vi "Factory_Acceptance_Test.vi"() -> ()   [LabVIEW 2020]
uses:
  <vilib>/Retry/UI Control Suite/Boolean/System Buttons/Graph Button.ctl
  Driver/E5071C/E5071C/E5071C.lvclass
  Driver/PEU/PEU/PEU.lvclass
  <vilib>/Utility/NIReport.llb/Report Type.ctl
  Driver/E5071C/E5071C/E5071C.lvclass/E5071C.ctl
  <vilib>/addons/_office/excel.llb/Excel Get Data ([str]).vi
  <vilib>/addons/_office/excel.llb/Excel Easy Table (str).vi
  <vilib>/Utility/NIReport.llb/NI_report.lvclass
  <instrlib>/Agilent ENA Series/Agilent ENA Series.lvlib
  <vilib>/Utility/NIReport.llb/NI_ReportGenerationCore.lvlib
  <vilib>/Utility/NIReport.llb/Excel/NI_Excel.lvclass
  <vilib>/addons/_office/NI_ReportGenerationToolkit.lvlib
panel:
  in  "Load":bool
  in  "Test":bool
  in  "Save":bool
  in  "负载选择":enum32{"Item 0", "Item 1"}(radio)
  in  "Limit Line":T1
  in  "DUT ID:":string
  in  "DUT\n开关类型":string(combo)="SPDT"
  in  "Panel Show":bool
  in  "Tab Control":enum32{"驻波VSWR", "插入损耗IL", "隔离度ISL"}(tab)
  out "VSWR_State":string
  out "VSWR Graph":cluster{"频率":dbl[], dbl[]}[](graph)
  out "IL_State":string
  out "IL Graph":cluster{"Freqs":dbl[], "temp_value":dbl[]}[](graph)
  out "ISL_State":string
  out "ISL Graph":cluster{"Freqs":dbl[], "temp_value":dbl[]}[](graph)
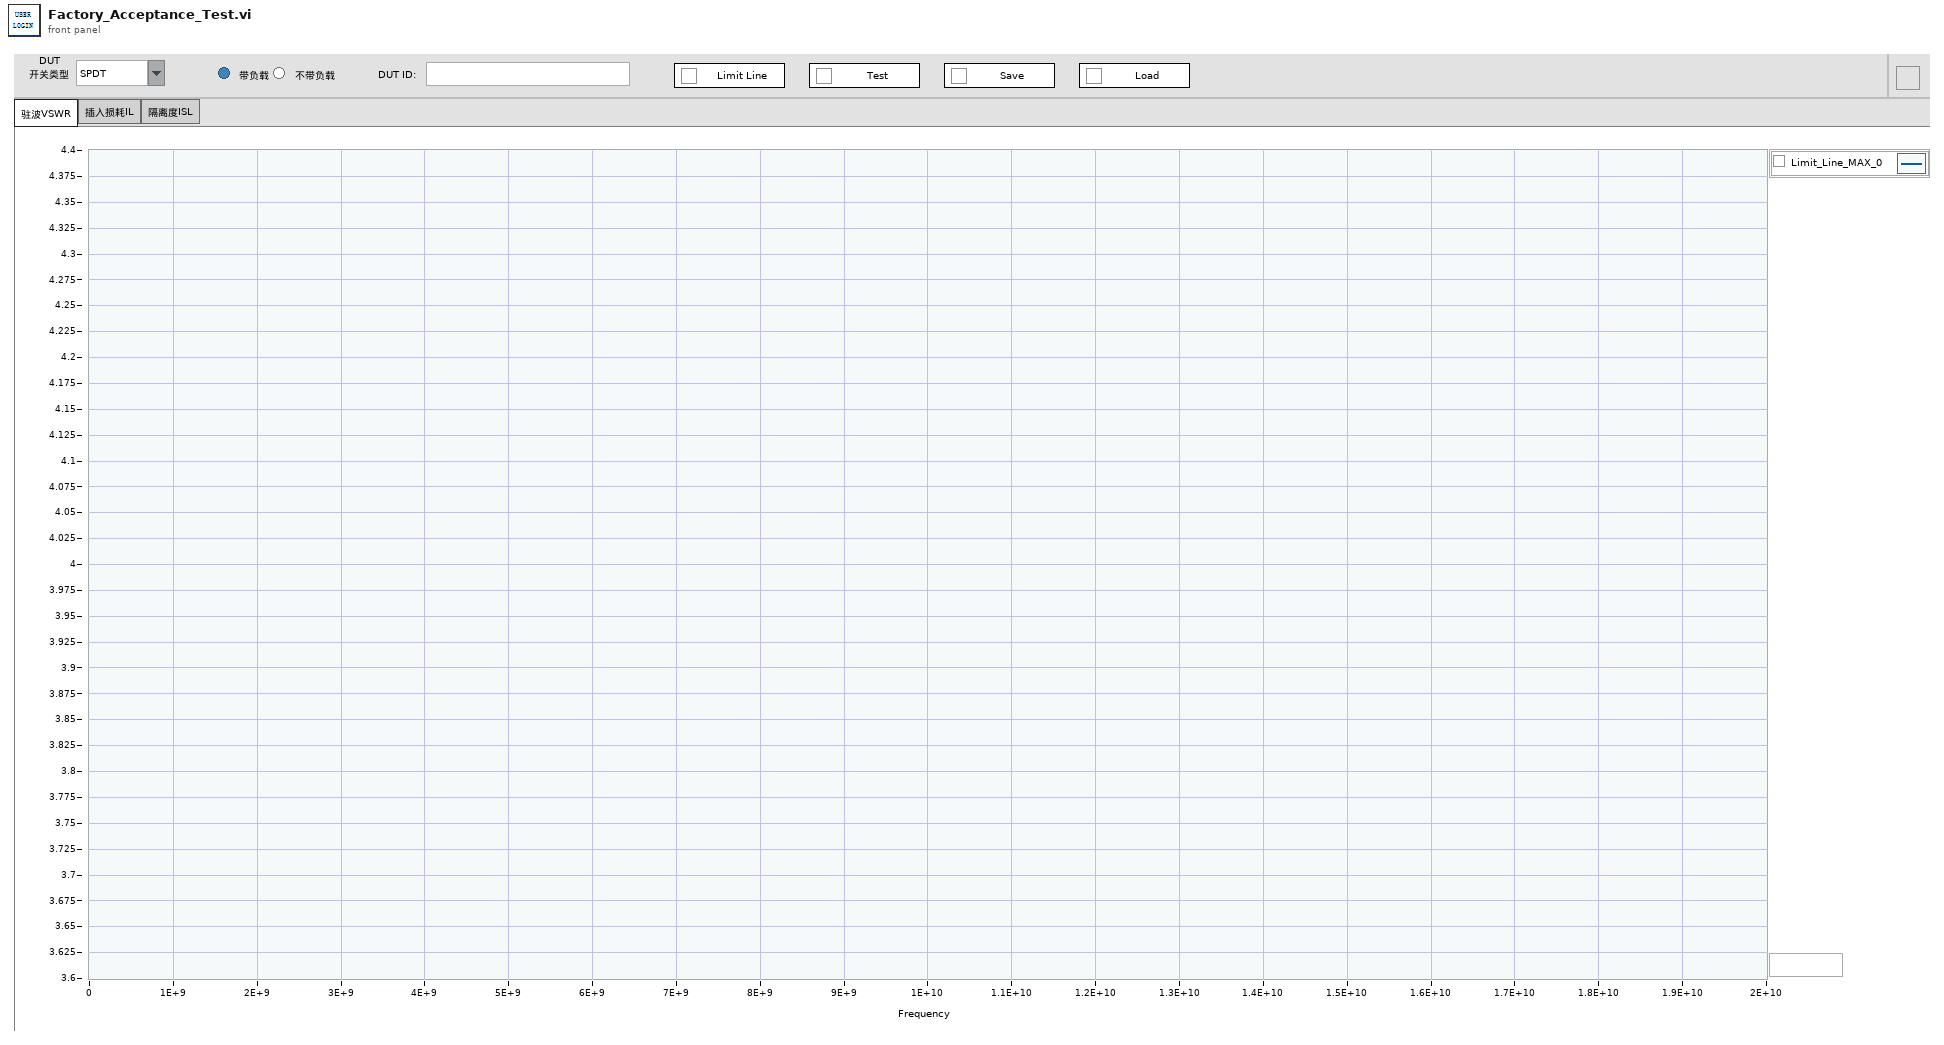
[diagram p1: front panel]
types:
  T1 = typedef "Graph Button.ctl" = bool
  T2 = enum32{"Invalid", "Standard", "Closed", "Hidden", "Minimized", "Maximized"}
  T3 = cluster{"Limit_IL":string[][], "Limit_VSWR":string[][], "Limit_ISL":string[][]}
  T4 = cluster{"校准文件":string[], "控制箱通道":string[], "DUT导通引脚":string[], "S名称":string[], "配置S":string[], "Plot_Name":string[]}
  T5 = typedef "NI_ReportGenerationCore.lvlib/Report Type.ctl" = enum16{"HTML", "Word", "Excel"}
  T6 = enum16{"maximized", "minimized", "normal", "no change"}
  T7 = cluster{"E5071C":refnum<class "E5071C.lvclass">, "PEU":refnum<class "PEU.lvclass">, "Index":i32, "Limit_Table":cluster{"Limit_IL":string[][], "Limit_VSWR":string[][], "Limit_ISL":string[][]}, "VSWR Graph":cluster{"频率":dbl[], dbl[]}[], "temp_value":dbl[], "Freqs":dbl[], "Count":i32, "测试逻辑":cluster{"校准文件":string[], "控制箱通道":string[], "DUT导通引脚":string[], "S名称":string[], "配置S":string[], "Plot_Name":string[]}, "VSWR_State":bool, "IL_State":bool, "ISL_State":bool, "Limit_Line_State":bool}
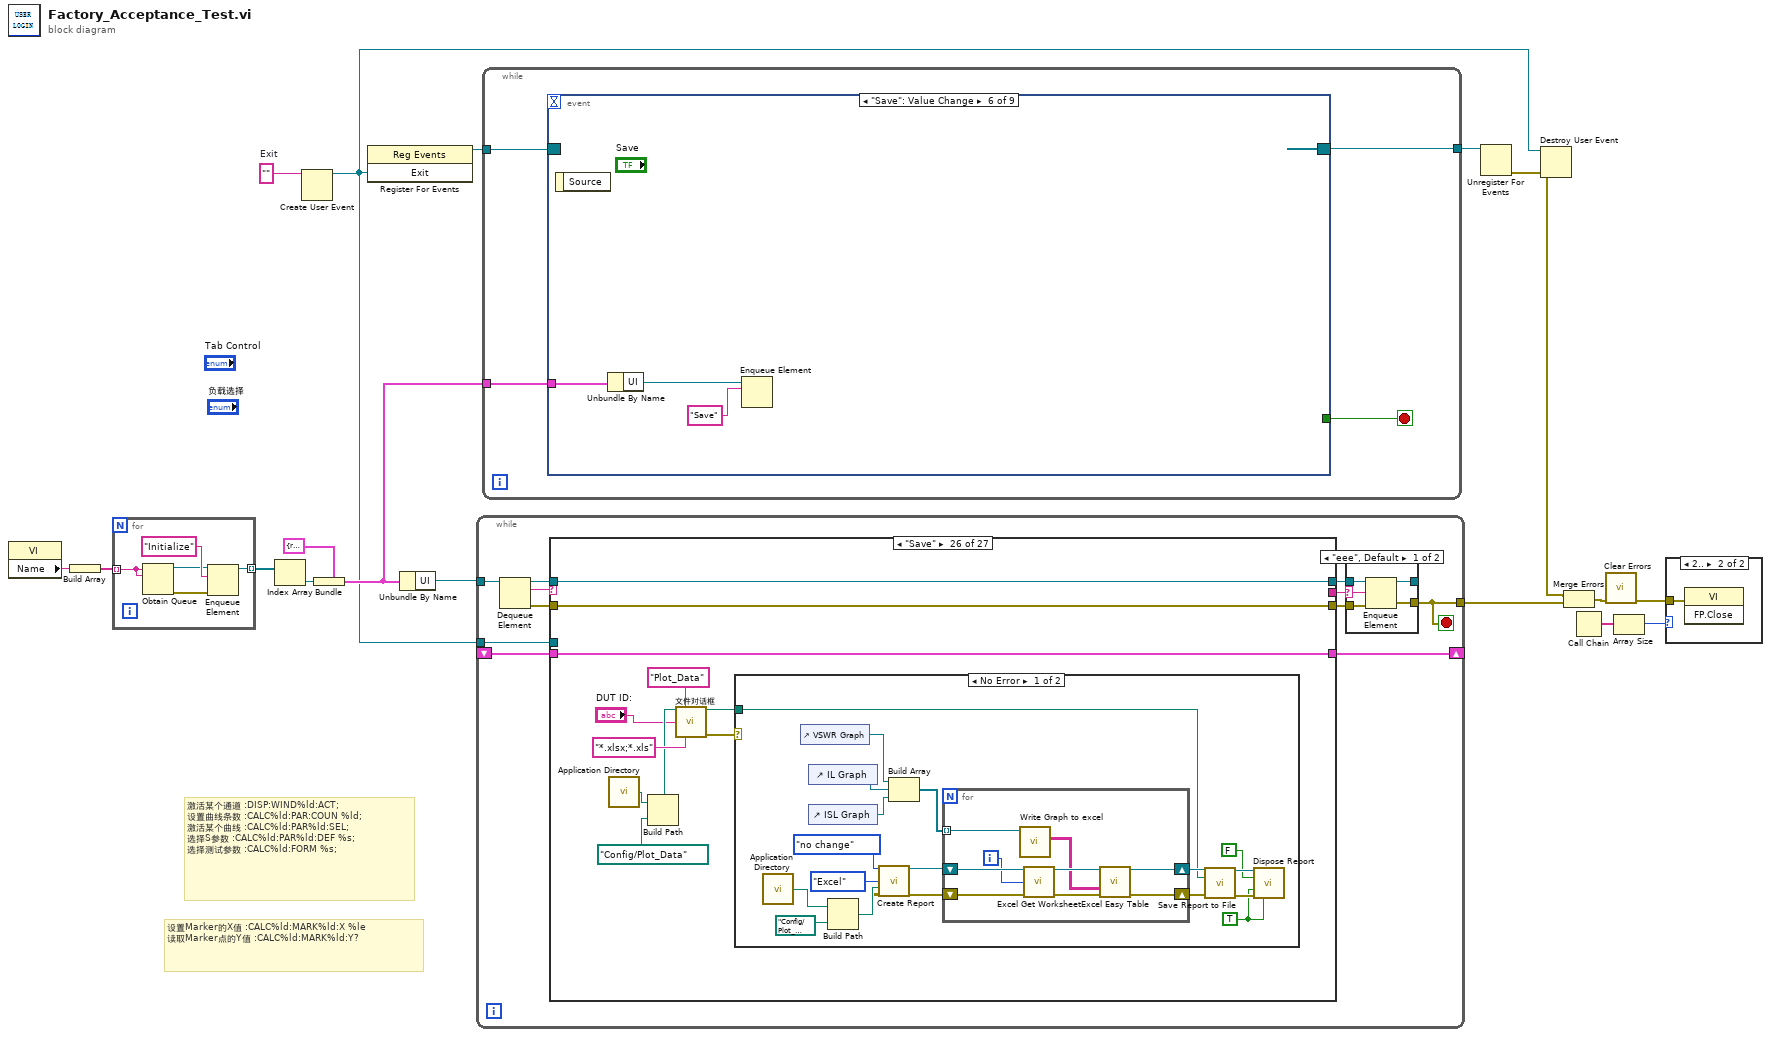
[diagram p0: block diagram]
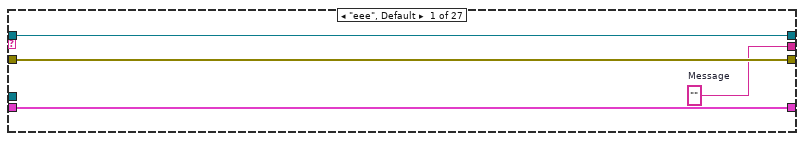
[diagram p4: hidden frame]
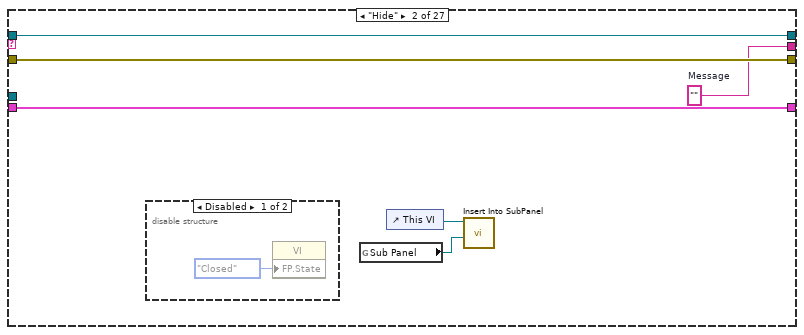
[diagram p5: hidden frame]
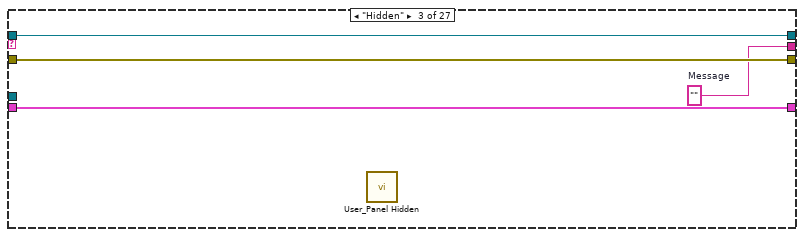
[diagram p7: hidden frame]
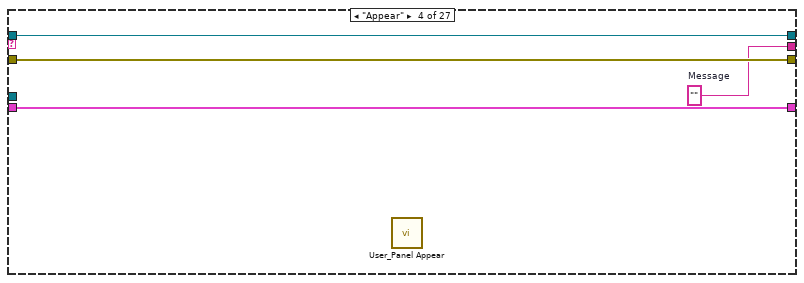
[diagram p8: hidden frame]
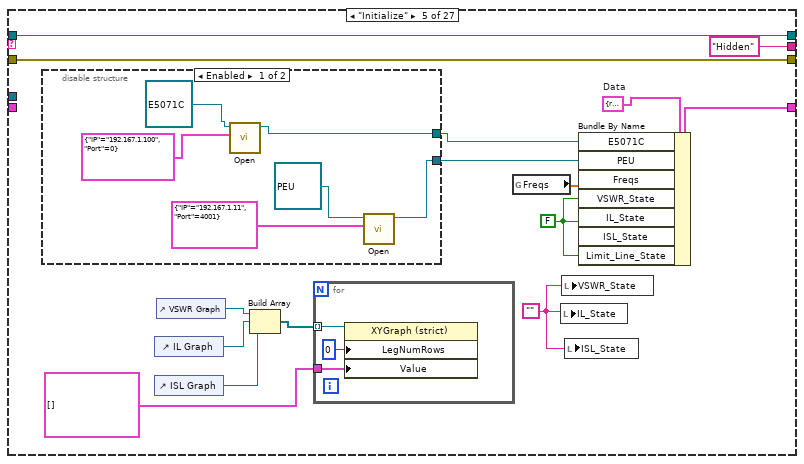
[diagram p9: hidden frame]
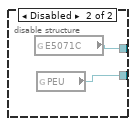
[diagram p10: hidden frame]
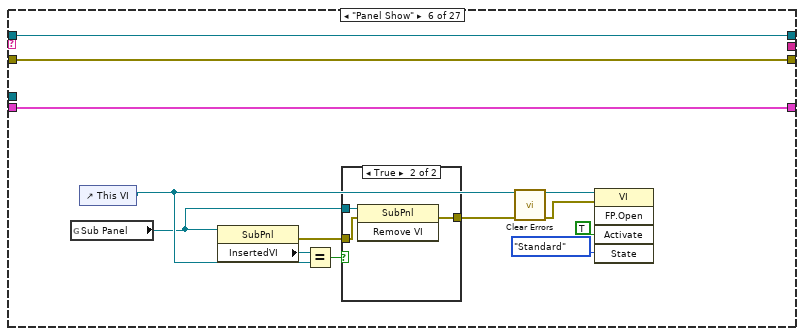
[diagram p11: hidden frame]
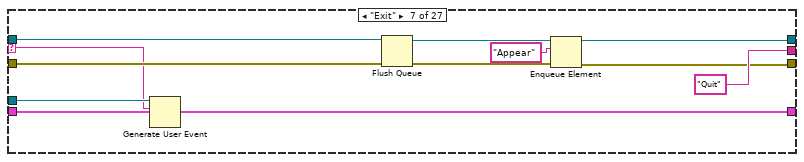
[diagram p13: hidden frame]
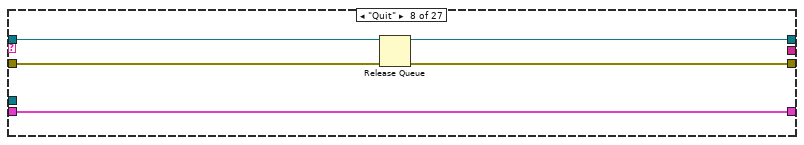
[diagram p14: hidden frame]
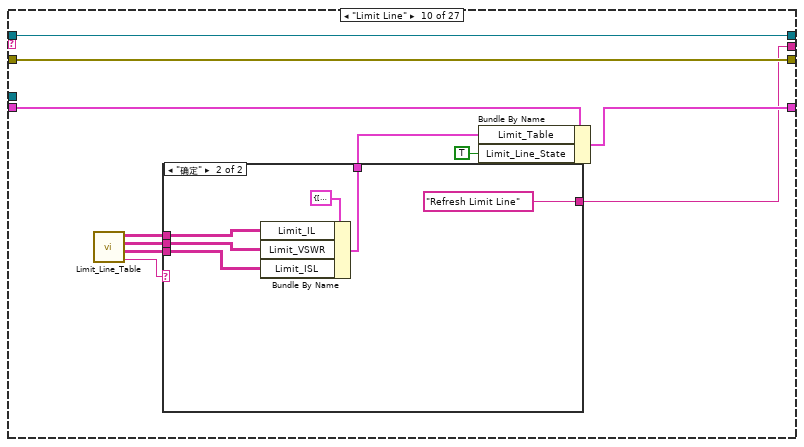
[diagram p16: hidden frame]
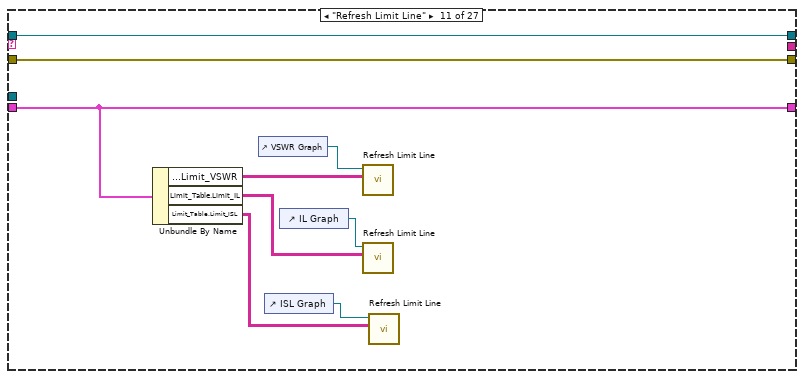
[diagram p18: hidden frame]
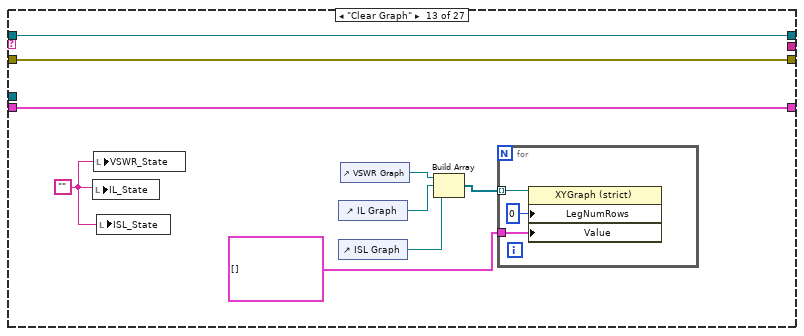
[diagram p20: hidden frame]
diagram:
  w7 = ""  # Exit
  # "设置Marker的X值\t:CALC%ld:MARK%ld:X %le\n读取Marker点的Y值\t:CALC%ld:MARK%ld:Y?"
  # "激活某个通道\t:DISP:WIND%ld:ACT;\n设置曲线条数\t:CALC%ld:PAR:COUN %ld;\n激活某个曲线\t:CALC%ld:PAR%ld:SEL;\n选择S参数\t:CALC%ld:PAR%ld:DEF %s;\n选择测试参数\t:CALC%ld:FORM %s;"
  n1 = property class="VI"() -> ("Name"=w17:string)  [unwired: 2 in, 2 out]
  n2 = Build Array(w17) -> (w18:string[])
  n3 = for {
    tunnel: w18 -> [w19] mode=indexing
    tunnel: [w20] -> w12 mode=indexing
    n4 = Obtain Queue(name (unnamed)=w19, element data type=w19) -> (queue out=w22:refnum<queue>, error out=w21:errorcluster)  [unwired: 3 in, 1 out]
    n5 = Enqueue Element(queue=w22, element="Initialize" ("元素"), error in (no error)=w21) -> (queue out=w20:refnum<queue>)  [unwired: 1 in, 2 out]
  }
  n6 = Index Array(array=w12) -> (element=w15:refnum<queue>)  [unwired: 1 in]
  n7 = Create User Event(user event datatype=w7) -> (user event=w11:refnum<user-event>)  [unwired: 1 in, 1 out]
  n8 = Bundle(cluster=cluster{"UI":refnum<queue>} {"UI"=refnum}, "UI"=w15) -> (w16:cluster{"UI":refnum<queue>})
  n9 = register-events(w11) -> (reference out=w8:refnum<event-registration>)  [unwired: 2 in, 1 out]
  n10 = Unbundle By Name(w16) -> ("UI"=w13:refnum<queue>)
  n11 = while {
    tunnel: w13 -> [w34]
    tunnel: [w24] -> w1
    shift-right: [w28] -> _
    shift-left: _ -> [w27]
    tunnel: w11 -> [w26]
    stop <- w24 stop-if-true
    n12 = Dequeue Element(queue=w34) -> (queue out=w33:refnum<queue>, element=w25:string, error out=w30:errorcluster)  [unwired: 2 in, 1 out]
    n13 = case shown="\"Save\"" w25 {
      selector: w25 -> [_ _ _ _ _ _ w107 _ _ _ _ _ _ _ _ _ _ _ _ _ _ _ _ _ _ _ _]
      tunnel: w33 -> [w45 w51 w56 w60 w75 w98 w110 w116 w119 w130 w145 w148 w157 w197 w206 w220 w232 w241 w253 w284 w319 w343 w374 w414 w418 w429 w463]
      tunnel: [w45 w51 w56 w60 w75 w98 w102 w116 w119 w130 w145 w148 w157 w197 w206 w220 w232 w241 w253 w284 w319 w343 w374 w414 w418 w429 w463] -> w32
      tunnel: [w44 w50 w55 w59 w74 w97 w103 w113 w117 w129 w144 w146 w155 w196 w205 w219 w231 w240 w252 w283 w318 w342 w373 w413 w416 w427 w462] -> w31
      tunnel: w30 -> [w44 w50 w55 w59 w74 w97 w109 w115 w117 w129 w144 w146 w155 w196 w205 w219 w231 w240 w252 w283 w318 w342 w373 w413 w416 w427 w462]
      tunnel: [w43 w49 w54 w58 "Hidden" ("Message") _ "Quit" ("Message") _ _ w121 _ _ _ "Judge_Condition" ("Message") w198 "Set_Control_Box" ("Message") "Set_Switch" ("Message") "Configure_S" ("Message") "Configure_Limit_Test" ("Message") "Measure_S" ("Message") "Refresh_Graph" ("Message") "Limit_State" "Judge_Condition" ("Message") _ _ _ _] -> w29
      tunnel: [w42 w48 w53 w57 w73 w96 w112 w114 w118 w122 w143 w147 w156 w191 w204 w209 w229 w238 w250 w281 w312 w338 w366 w410 w417 w428 w461] -> w28
      tunnel: w27 -> [w42 w48 w53 w57 _ w96 w112 w114 w118 w124 w143 w147 w156 w192 w204 w209 w229 w238 w250 w281 w313 w338 w365 w412 w417 w428 w461]
      tunnel: w26 -> [_ _ _ _ _ _ w108 _ _ _ _ _ _ _ _ _ _ _ _ _ _ _ _ _ _ _ _]
      frame "eee", Default {
        w43 = ""  # Message
      }
      frame "Hide" {
        w49 = ""  # Message
        n14 = disable-structure shown="Disabled" {
          frame Disabled {
            n15 = property class="VI"("FP.State"=T2."Closed" ("前面板窗口:状态")) -> ()  [unwired: 2 in, 2 out]
          }
          frame Enabled {
          }
        }
        n16 = global read "Global.vi" "Sub Panel"() -> (w46:refnum<vi>)
        n17 = control-ref of="This VI"() -> (w47:refnum<vi>)
        n18 = call "Insert Into SubPanel.vi"("SubPanel Ref"=w46, "VI Ref In"=w47) -> ()  [unwired: 9 in, 1 out]
      }
      frame "Hidden" {
        w54 = ""  # Message
        n19 = call "User_Panel Hidden.vi"() -> ()  [unwired: 11 in, 1 out]
      }
      frame "Appear" {
        w58 = ""  # Message
        n20 = call "User_Panel Appear.vi"() -> ()  [unwired: 11 in, 1 out]
      }
      frame "Initialize" {
        w67 = T7 {"E5071C"=refnum, "PEU"=refnum, "Index"=0, "Limit_Table"={"Limit_IL"=[], "Limit_VSWR"=[], "Limit_ISL"=[]}, "VSWR Graph"=[], "temp_value"=[], "Freqs"=[], "Count"=0, "测试逻辑"={"校准文件"=[], "控制箱通道"=[], "DUT导通引脚"=[], "S名称"=[], "配置S"=[], "Plot_Name"=[]}, "VSWR_State"=FALSE, "IL_State"=FALSE, "ISL_State"=FALSE, "Limit_Line_State"=FALSE}  # Data
        w68 = ""
        w66 = FALSE
        n21 = disable-structure shown="Enabled" {
          disable-tunnel: [w79 w86] -> w70
          disable-tunnel: [w83 w85] -> w69
          frame Enabled {
            n22 = call "Open.vi"("Link"=cluster{"IP":string, "Port":u32} {"IP"="192.167.1.100", "Port"=0}, "E5071C in"=refnum<class "E5071C.lvclass"> refnum ("E5071C.lvlib:E5071C.lvclass")) -> ("E5071C out"=w79:refnum<class "E5071C.lvclass">)  [unwired: 7 in, 2 out]
            n23 = call "Open.vi"("Link"=cluster{"IP":string, "Port":u16} {"IP"="192.167.1.11", "Port"=4001}, "PEU in"=refnum<class "PEU.lvclass"> refnum ("PEU.lvlib:PEU.lvclass")) -> ("PEU out"=w83:refnum<class "PEU.lvclass">)  [unwired: 7 in, 2 out]
          }
          frame Disabled {
            n24 = global read "Global.vi" "E5071C"() -> (w86:refnum<class "E5071C.lvclass">)
            n25 = global read "Global.vi" "PEU"() -> (w85:refnum<class "PEU.lvclass">)
          }
        }
        n26 = control-ref of="IL Graph"() -> (w63:refnum<vi>)
        n27 = control-ref of="ISL Graph"() -> (w64:refnum<vi>)
        n28 = control-ref of="VSWR Graph"() -> (w62:refnum<vi>)
        n29 = Build Array(w62, w63, w64) -> (w65:refnum<vi>[])
        n30 = for {
          tunnel: w65 -> [w77] mode=indexing
          tunnel: cluster{"频率":dbl[], dbl[]}[] [] ("VSWR Graph") -> [w76]
          n31 = property class="XYGraph (strict)"(reference=w77, "LegNumRows"=u32 0 ("Legend:Number of Rows"), "Value"=w76) -> ()  [unwired: 1 in, 2 out]
        }
        n32 = global read "Global.vi" "Freqs"() -> (w71:dbl[])
        n33 = local write "IL_State"(w68) -> ()
        n34 = local write "VSWR_State"(w68) -> ()
        n35 = local write "ISL_State"(w68) -> ()
        n36 = Bundle By Name(cluster=w67, "E5071C"=w70, "PEU"=w69, "Freqs"=w71, "VSWR_State"=w66, "IL_State"=w66, "ISL_State"=w66, "Limit_Line_State"=w66) -> (w73:T7)
      }
      frame "Panel Show" {
        n37 = global read "Global.vi" "Sub Panel"() -> (w87:refnum<vi>)
        n38 = control-ref of="This VI"() -> (w88:refnum<vi>)
        n39 = property class="SubPnl"(reference=w87) -> (error out=w95:errorcluster, "InsertedVI"=w93:refnum<vi>)  [unwired: 1 in, 1 out]
        n40 = Equal?(x=w93, y=w88) -> (x = y?=w94:bool)
        n41 = case shown="True" w94 {
          tunnel: [_ w101] -> w89
          tunnel: w87 -> [_ w100]
          tunnel: w95 -> [_ w99]
          frame False {
          }
          frame True {
            n42 = invoke class="SubPnl" method="Remove VI"(reference=w100, error in=w99) -> (error out=w101:errorcluster)  [unwired: 1 in, 2 out]
          }
        }
        n43 = call <vilib>:"Clear Errors.vi"("error in (no error)"=w89) -> ("error out"=w92:errorcluster)  [unwired: 5 in, 1 out]
        n44 = invoke class="VI" method="FP.Open"(reference=w88, error in=w92, "Activate"=TRUE ("激活？"), "State"=T2."Standard" ("状态")) -> ()  [unwired: 1 in, 5 out]
      }
      frame "Exit" {
        n45 = Generate User Event(user event=w108, event data cluster=w107) -> ()  [unwired: 2 in, 2 out]
        n46 = Flush Queue(queue=w110, error in (no error)=w109) -> (queue out=w105:refnum<queue>, error out=w104:errorcluster)  [unwired: 1 out]
        n47 = Enqueue Element(queue=w105, element="Appear" ("元素"), error in (no error)=w104) -> (queue out=w102:refnum<queue>, error out=w103:errorcluster)  [unwired: 1 in, 1 out]
      }
      frame "Quit" {
        n48 = Release Queue(queue=w116, error in (no error)=w115) -> (error out=w113:errorcluster)  [unwired: 1 in, 2 out]
      }
      frame "----------------------Limit Line----------------" {
      }
      frame "Limit Line" {
        n49 = call "Limit_Line_Table.vi"() -> ("状态"=w125:string, "Limit_ISL"=w126:string[][], "Limit_VSWR"=w127:string[][], "Limit_IL"=w128:string[][])  [unwired: 8 in]
        n50 = case shown="\"确定\"" w125 {
          tunnel: w128 -> [_ w135]
          tunnel: w127 -> [_ w132]
          tunnel: w126 -> [_ w134]
          tunnel: [_ w133] -> w123
          tunnel: [_ "Refresh Limit Line" ("Message")] -> w121
          frame "取消", Default {
          }
          frame "确定" {
            n51 = Bundle By Name(cluster=T3 {"Limit_IL"=[], "Limit_VSWR"=[], "Limit_ISL"=[]} ("Limit_Table"), "Limit_IL"=w135, "Limit_VSWR"=w132, "Limit_ISL"=w134) -> (w133:T3)
          }
        }
        n52 = Bundle By Name(cluster=w124, "Limit_Table"=w123, "Limit_Line_State"=TRUE) -> (w122:T7)
      }
      frame "Refresh Limit Line" {
        n53 = Unbundle By Name(w143) -> ("Limit_Table.Limit_VSWR"=w141:string[][], "Limit_Table.Limit_IL"=w140:string[][], "Limit_Table.Limit_ISL"=w138:string[][])
        n54 = control-ref of="VSWR Graph"() -> (w142:refnum<vi>)
        n55 = control-ref of="ISL Graph"() -> (w137:refnum<vi>)
        n56 = control-ref of="IL Graph"() -> (w139:refnum<vi>)
        n57 = call "Refresh Limit Line.vi"("Item Names"=w141, "XY Graph"=w142) -> ()  [unwired: 9 in, 1 out]
        n58 = call "Refresh Limit Line.vi"("Item Names"=w140, "XY Graph"=w139) -> ()  [unwired: 9 in, 1 out]
        n59 = call "Refresh Limit Line.vi"("Item Names"=w138, "XY Graph"=w137) -> ()  [unwired: 9 in, 1 out]
      }
      frame "------------Measurement----------" {
      }
      frame "Clear Graph" {
        w154 = ""
        n60 = local write "IL_State"(w154) -> ()
        n61 = local write "VSWR_State"(w154) -> ()
        n62 = local write "ISL_State"(w154) -> ()
        n63 = control-ref of="IL Graph"() -> (w151:refnum<vi>)
        n64 = control-ref of="ISL Graph"() -> (w152:refnum<vi>)
        n65 = control-ref of="VSWR Graph"() -> (w150:refnum<vi>)
        n66 = Build Array(w150, w151, w152) -> (w153:refnum<vi>[])
        n67 = for {
          tunnel: w153 -> [w159] mode=indexing
          tunnel: cluster{"频率":dbl[], dbl[]}[] [] ("VSWR Graph") -> [w158]
          n68 = property class="XYGraph (strict)"(reference=w159, "LegNumRows"=u32 0 ("Legend:Number of Rows"), "Value"=w158) -> ()  [unwired: 1 in, 2 out]
        }
      }
      frame "Read_Switch_excel" {
        n69 = call <vilib>:"Application Directory.vi"() -> ("Application Directory"=w194:path)
        n70 = Build Path(base path=w194, name or relative path=path "Config/开关映射表.xlsx") -> (appended path=w190:path)
        n71 = call <vilib>:"Create Report.vi"("window state (normal)"=T6."no change", "report type"=Report_Type."Excel", "template (empty)"=w190) -> ("report out"=w187:refnum<class "NI_report.lvclass">, "error out"=w186:errorcluster)  [unwired: 11 in]
        n72 = call <vilib>:"Excel Get Worksheet.vi"("report in"=w187, "error in (no error)"=w186, "name (\"\")"="DUT\n开关类型") -> ("report out"=w184:refnum<class "NI_report.lvclass">, "error out"=w183:errorcluster)  [unwired: 11 in]
        n73 = call-poly <vilib>:"Excel Get Data.vi"("report in"=w184, "data type"=string[][] [], "error in (no error)"=w183) -> ("report out"=w163:refnum<class "NI_report.lvclass">, "data"=w167:string[][], "error out"=w162:errorcluster)  [unwired: 10 in]
        n74 = Delete From Array(array=w167, index (row)=0) -> (array with subset deleted=w179:string[][])  [unwired: 2 in, 1 out]
        n75 = call-dynamic "Dispose Report.vi"("report in"=w163, "error in (no error)"=w162) -> ()  [unwired: 13 in, 1 out]
        n76 = Index Array(array=w179, index (col) #1=0 ("disabled index (col)"), index (col) #2=1 ("disabled index (col)"), index (col) #3=2 ("disabled index (col)"), index (col) #4=3 ("disabled index (col)"), index (col) #5=4 ("disabled index (col)"), index (col) #6=5 ("disabled index (col)")) -> (element #1=w166:string[], element #2=w172:string[], element #3=w171:string[], element #4=w170:string[], element #5=w169:string[], element #6=w168:string[])  [unwired: 6 in]
        n77 = Array Size(array=w166) -> (size(s)=w165:i32)
        n78 = Bundle By Name(cluster=T4 {"校准文件"=[], "控制箱通道"=[], "DUT导通引脚"=[], "S名称"=[], "配置S"=[], "Plot_Name"=[]}, "校准文件"=w166, "控制箱通道"=w172, "DUT导通引脚"=w171, "S名称"=w170, "配置S"=w169, "Plot_Name"=w168) -> (w164:T4)
        n79 = Bundle By Name(cluster=w192, "Index"=0, "Count"=w165, "测试逻辑"=w164) -> (w191:T7)
      }
      frame "Judge_Condition" {
        n80 = Unbundle By Name(w204) -> ("Index"=w203:i32, "Count"=w202:i32)
        n81 = Equal?(x=w203, y=w202) -> (x = y?=w201:bool)
        n82 = Select(t="End_Test", s=w201, f="Load_Calibration_File" ("Message")) -> (s? t:f=w198:string)
      }
      frame "Load_Calibration_File" {
        n83 = Unbundle By Name(w209) -> ("E5071C"=w217:refnum<class "E5071C.lvclass">, "测试逻辑.校准文件"=w211:string[], "Index"=w210:i32)
        n84 = Index Array(array=w211, index=w210) -> (element=w207:string)
        n85 = Concatenate Strings("XK/", w207, ".sta") -> (w214:string)
        n86 = Format Into String(format string=":MMEM:LOAD \"%s\"" ("Command"), w214) -> (resulting string=w212:string)  [unwired: 2 in, 1 out]
        n87 = call "Query.vi"("Return"=FALSE, "Command"=w212, "E5071C in"=w217) -> ()  [unwired: 6 in, 3 out]
      }
      frame "Set_Control_Box" {
        n88 = Unbundle By Name(w229) -> ("PEU"=w228:refnum<class "PEU.lvclass">, "测试逻辑.控制箱通道"=w227:string[], "Index"=w226:i32)
        n89 = Index Array(array=w227, index=w226) -> (element=w225:string)
        n90 = call <vilib>:"Delimited String to 1D String Array.vi"("delimiter"=",", "delimited string"=w225) -> ("string array"=w223:string[])  [unwired: 9 in]
        n91 = Index Array(array=w223) -> (element #1=w222:string, element #2=w221:string)  [unwired: 2 in]
        n92 = call "Switch Channel.vi"("CH2"=w221, "CH1"=w222, "PEU in"=w228) -> ()  [unwired: 7 in, 2 out]
      }
      frame "Set_Switch" {
        n93 = Unbundle By Name(w238) -> ("PEU"=w235:refnum<class "PEU.lvclass">, "测试逻辑.DUT导通引脚"=w237:string[], "Index"=w236:i32)
        n94 = Index Array(array=w237, index=w236) -> (element=w234:string)
        n95 = Decimal String To Number(string=w234) -> (number=w233:i32)  [unwired: 2 in, 1 out]
        n96 = call "Set Switch Pin High.vi"("Pin"=w233, "PEU in"=w235) -> ()  [unwired: 8 in, 2 out]
      }
      frame "Configure_S" {
        n97 = Unbundle By Name(w250) -> ("E5071C"=w249:refnum<class "E5071C.lvclass">, "测试逻辑.配置S"=w245:string[], "Index"=w244:i32)
        n98 = Index Array(array=w245, index=w244) -> (element=w243:string)
        n99 = call "Read E5071C_VISA.vi"("E5071C in"=w249) -> ("E5071C_VISA"=w248:refnum<visa-resource-name>)  [unwired: 8 in, 2 out]
        n100 = case shown="\"S21\"" w243 {
          tunnel: [w255 w256 w259] -> w247
          tunnel: [w254 w257 w258] -> w246
          frame "S11", Default {
            w255 = u16 12 items=["Logarithmic Magnitude", "Phase", "Group Delay", "Smith Chart  Linear (Lin/Phase)", "Smith Chart  Logarithmic (Log/Phase)", "Smith Chart  Complex (Real/Imag)", "Smith Chart  Impedance (R+jX)", "Smith Chart  Admittance (G+jB)", "Polar Format (Linear)", "Polar Format (Logarithmic)", "Polar Format (Re/Im)", "Linear Magnitude", "SWR", "Real", "Imaginary", "Epanded Phase", "Positive Phase"] ("Data Format (0: Logarithmic Magnitude)")
            w254 = u16 0 items=["S11", "S21", "S31", "S41", "S12", "S22", "S32", "S42", "S13", "S23", "S33", "S43", "S14", "S24", "S34", "S44", "A", "B", "C", "D", "R1", "R2", "R3", "R4", "AUX1", "AUX2", "TR", "T", "R"] ("Measurement Parameters (0: S11)")
            # "S11"
          }
          frame "S21" {
            w256 = u16 0 items=["Logarithmic Magnitude", "Phase", "Group Delay", "Smith Chart  Linear (Lin/Phase)", "Smith Chart  Logarithmic (Log/Phase)", "Smith Chart  Complex (Real/Imag)", "Smith Chart  Impedance (R+jX)", "Smith Chart  Admittance (G+jB)", "Polar Format (Linear)", "Polar Format (Logarithmic)", "Polar Format (Re/Im)", "Linear Magnitude", "SWR", "Real", "Imaginary", "Epanded Phase", "Positive Phase"] ("Data Format (0: Logarithmic Magnitude)")
            w257 = u16 1 items=["S11", "S21", "S31", "S41", "S12", "S22", "S32", "S42", "S13", "S23", "S33", "S43", "S14", "S24", "S34", "S44", "A", "B", "C", "D", "R1", "R2", "R3", "R4", "AUX1", "AUX2", "TR", "T", "R"] ("Measurement Parameters (0: S11)")
            # "S21(IL)"
          }
          frame "S22" {
            w259 = u16 12 items=["Logarithmic Magnitude", "Phase", "Group Delay", "Smith Chart  Linear (Lin/Phase)", "Smith Chart  Logarithmic (Log/Phase)", "Smith Chart  Complex (Real/Imag)", "Smith Chart  Impedance (R+jX)", "Smith Chart  Admittance (G+jB)", "Polar Format (Linear)", "Polar Format (Logarithmic)", "Polar Format (Re/Im)", "Linear Magnitude", "SWR", "Real", "Imaginary", "Epanded Phase", "Positive Phase"] ("Data Format (0: Logarithmic Magnitude)")
            w258 = u16 5 items=["S11", "S21", "S31", "S41", "S12", "S22", "S32", "S42", "S13", "S23", "S33", "S43", "S14", "S24", "S34", "S44", "A", "B", "C", "D", "R1", "R2", "R3", "R4", "AUX1", "AUX2", "TR", "T", "R"] ("Measurement Parameters (0: S11)")
            # "S22"
          }
        }
        n101 = call <instrlib>:"Configure Channel And Trace.vi"("Data Format (0: Logarithmic Magnitude)"=w247, "Measurement Parameters (0: S11)"=w246, "VISA resource name"=w248) -> ()  [unwired: 7 in, 2 out]
        n102 = Wait (ms)(milliseconds to wait=u32 2000) -> ()  [unwired: 1 out]
      }
      frame "Configure_Limit_Test" {
        n103 = Unbundle By Name(w281) -> ("测试逻辑.S名称"=w264:string[], "Index"=w263:i32, "Limit_Table"=w267:T3, "E5071C"=w265:refnum<class "E5071C.lvclass">, "Limit_Line_State"=w260:bool)
        n104 = Index Array(array=w264, index=w263) -> (element=w262:string)
        n105 = case shown="\"驻波\", Default" w262 {
          tunnel: w267 -> [w301 w303 w305]
          tunnel: [w300 w302 w304] -> w266
          frame "驻波", Default {
            n106 = Unbundle By Name(w301) -> ("Limit_VSWR"=w300:string[][])
          }
          frame "插损" {
            n107 = Unbundle By Name(w303) -> ("Limit_IL"=w302:string[][])
          }
          frame "隔离" {
            n108 = Unbundle By Name(w305) -> ("Limit_ISL"=w304:string[][])
          }
        }
        n109 = Index Array(array=w266, index (col) #1=1 ("disabled index (col)"), index (col) #2=2 ("index (col)"), index (col) #3=3 ("index (col)"), index (col) #4=4 ("index (col)"), index (col) #5=5 ("index (col)")) -> (element #1=w279:string[], element #2=w276:string[], element #3=w273:string[], element #4=w269:string[], element #5=w268:string[])  [unwired: 5 in]
        n110 = Matrix Size(0:w266) -> (1:w261:i32)  [unwired: 1 out]
        n111 = Fract/Exp String To Number(string=w276) -> (number=w275:dbl[])  [unwired: 3 in, 1 out]
        n112 = Fract/Exp String To Number(string=w273) -> (number=w272:dbl[])  [unwired: 3 in, 1 out]
        n113 = for {
          tunnel: w279 -> [w307] mode=indexing
          tunnel: [w306] -> w278 mode=indexing
          n114 = case shown="\"OFF\", Default" w307 {
            tunnel: [0 1 2] -> w306
            frame "OFF", Default {
            }
            frame "MAX" {
            }
            frame "MIN" {
            }
          }
        }
        n115 = case shown="True" w260 {
          tunnel: w278 -> [_ w295]
          tunnel: w275 -> [_ w294]
          tunnel: w272 -> [_ w293]
          tunnel: w269 -> [_ w292]
          tunnel: w268 -> [_ w290]
          tunnel: w265 -> [_ w288]
          tunnel: w261 -> [_ w286]
          frame False {
          }
          frame True {
            n116 = call "Read E5071C_VISA.vi"("E5071C in"=w288) -> ("E5071C_VISA"=w299:refnum<visa-resource-name>)  [unwired: 8 in, 2 out]
            n117 = call <instrlib>:"Configure Limit Test.vi"("Limit Line Display (F: Disable)"=TRUE, "Limit Test (F: Disable)"=TRUE, "Limit Fail Display (F: Disable)"=TRUE, "VISA resource name"=w299) -> ("error out"=w296:errorcluster, "VISA resource name out"=w297:refnum<visa-resource-name>)  [unwired: 6 in]
            n118 = Fract/Exp String To Number(string=w290) -> (number=w289:dbl[])  [unwired: 3 in, 1 out]
            n119 = Fract/Exp String To Number(string=w292) -> (number=w291:dbl[])  [unwired: 3 in, 1 out]
            n120 = call <instrlib>:"Configure Limit Test Table.vi"("VISA resource name"=w297, "Number of Lines (0)"=w286, "Type of Line (0)"=w295, "Start Point X Value (0.0)"=w294, "End Point X Value (0.0)"=w293, "error in (no error)"=w296, "Start Point Y Value (0.0)"=w291, "End Point Y Value (0.0)"=w289) -> ()  [unwired: 6 in, 2 out]
          }
        }
      }
      frame "Measure_S" {
        n121 = Unbundle By Name(w313) -> ("E5071C"=w316:refnum<class "E5071C.lvclass">, "Freqs"=w314:dbl[])
        n122 = call "Read E5071C_VISA.vi"("E5071C in"=w316) -> ("E5071C_VISA"=w315:refnum<visa-resource-name>)  [unwired: 8 in, 2 out]
        n123 = for {
          tunnel: w315 -> [w322]
          tunnel: w314 -> [w321] mode=indexing
          tunnel: [w320] -> w311 mode=indexing
          n124 = call <instrlib>:"Set Marker Position.vi"("X Value (0.0)"=w321, "VISA resource name"=w322) -> ("error out"=w323:errorcluster, "VISA resource name out"=w324:refnum<visa-resource-name>)  [unwired: 8 in]
          n125 = call <instrlib>:"Marker Data.vi"("error in (no error)"=w323, "VISA resource name"=w324) -> ("Y Real Value"=w320:dbl)  [unwired: 5 in, 4 out]
        }
        n126 = Bundle By Name(cluster=w313, "temp_value"=w311) -> (w312:T7)
      }
      frame "Refresh_Graph" {
        n127 = Unbundle By Name(w338) -> ("测试逻辑.S名称"=w340:string[], "Index"=w330:i32, "Freqs"=w328:dbl[], "temp_value"=w327:dbl[], "测试逻辑.Plot_Name"=w331:string[])
        n128 = Index Array(array=w340, index=w330) -> (element=w339:string)
        n129 = Index Array(array=w331, index=w330) -> (element=w329:string)
        n130 = Bundle("Freqs"=w328, "temp_value"=w327) -> (w326:cluster{"Freqs":dbl[], "temp_value":dbl[]})  [unwired: 1 in]
        n131 = case shown="\"隔离\"" w339 {
          tunnel: [w346 w351 w357] -> w332
          tunnel: w326 -> [w345 w353 w359]
          tunnel: [enum32{"驻波VSWR", "插入损耗IL", "隔离度ISL"}."驻波VSWR" ("Tab Control") enum32{"驻波VSWR", "插入损耗IL", "隔离度ISL"}."插入损耗IL" ("Tab Control") enum32{"驻波VSWR", "插入损耗IL", "隔离度ISL"}."隔离度ISL" ("Tab Control")] -> w325
          frame "驻波", Default {
            # "S11、S22"
            n132 = control-ref of="VSWR Graph"() -> (w348:refnum<vi>)
            n133 = property class="XYGraph (strict)"(reference=w348) -> (reference out=w346:refnum<vi>, "Value"=w347:cluster{"频率":dbl[], dbl[]}[])  [unwired: 1 in, 1 out]
            n134 = Build Array (concatenate)(w347, w345) -> (→"VSWR Graph":cluster{"Freqs":dbl[], "temp_value":dbl[]}[])
          }
          frame "插损" {
            # "S21(IL)"
            n135 = control-ref of="IL Graph"() -> (w355:refnum<vi>)
            n136 = property class="XYGraph (strict)"(reference=w355) -> (reference out=w351:refnum<vi>, "Value"=w354:cluster{"Freqs":dbl[], "temp_value":dbl[]}[])  [unwired: 1 in, 1 out]
            n137 = Build Array (concatenate)(w354, w353) -> (→"IL Graph":cluster{"Freqs":dbl[], "temp_value":dbl[]}[])
          }
          frame "隔离" {
            # "S21(ISO)"
            n138 = control-ref of="ISL Graph"() -> (w361:refnum<vi>)
            n139 = property class="XYGraph (strict)"(reference=w361) -> (reference out=w357:refnum<vi>, "Value"=w360:cluster{"Freqs":dbl[], "temp_value":dbl[]}[])  [unwired: 1 in, 1 out]
            n140 = Build Array (concatenate)(w360, w359) -> (→"ISL Graph":cluster{"Freqs":dbl[], "temp_value":dbl[]}[])
          }
        }
        n141 = local write "Tab Control"(w325) -> ()
        n142 = property class="XYGraph (strict)"(reference=w332) -> (reference out=w337:refnum<vi>, "LegNumRows"=w335:u32)  [unwired: 1 in, 1 out]
        n143 = Increment(x=w335) -> (x+1=w336:u32)
        n144 = property class="XYGraph (strict)"(reference=w337, "LegNumRows"=w336, "Active Plot"=w335, "Plot.Plot Name"=w329, "Plot.Line Width"=u8 2, "Plot.Visible?"=TRUE ("Plot.Visible")) -> ()  [unwired: 1 in, 2 out]
      }
      frame "Limit_State" {
        n145 = Unbundle By Name(w365) -> ("测试逻辑.S名称"=w369:string[], "Index"=w364:i32, "E5071C"=w372:refnum<class "E5071C.lvclass">)
        n146 = Increment(x=w364) -> (x+1=w363:i32)
        n147 = call "Read E5071C_VISA.vi"("E5071C in"=w372) -> ("E5071C_VISA"=w371:refnum<visa-resource-name>)  [unwired: 8 in, 2 out]
        n148 = Bundle By Name(cluster=w365, "Index"=w363) -> (w362:T7)
        n149 = call <instrlib>:"Limit Fail.vi"("VISA resource name"=w371) -> ("Limit Fail"=w367:bool)  [unwired: 8 in, 2 out]
        n150 = Index Array(array=w369, index=w364) -> (element=w368:string)
        n151 = case shown="\"隔离\"" w368 {
          tunnel: w367 -> [w384 w395 w406]
          tunnel: w362 -> [w381 w392 w403]
          tunnel: [w380 w391 w402] -> w366
          frame "驻波", Default {
            n152 = Unbundle By Name(w381) -> ("VSWR_State"=w385:bool)
            n153 = Or(x=w385, y=w384) -> (x .or. y?=w377:bool)
            n154 = Bundle By Name(cluster=w381, "VSWR_State"=w377) -> (w380:T7)
            n155 = Select(t=u32 16711680 ("Text.Text Colors:Text Color"), s=w377, f=u32 6618880 ("Text.Text Colors:Text Color")) -> (s? t:f=w375:u32)
            n156 = Select(t="FAIL", s=w377, f="PASS") -> (s? t:f=→"VSWR_State":string)
            n157 = property on="VSWR_State" class="Str"("Text.TextColor"=w375) -> ()  [unwired: 2 in, 2 out]
          }
          frame "插损" {
            n158 = Unbundle By Name(w392) -> ("IL_State"=w396:bool)
            n159 = Or(x=w396, y=w395) -> (x .or. y?=w388:bool)
            n160 = Bundle By Name(cluster=w392, "IL_State"=w388) -> (w391:T7)
            n161 = Select(t=u32 16711680 ("Text.Text Colors:Text Color"), s=w388, f=u32 6618880 ("Text.Text Colors:Text Color")) -> (s? t:f=w386:u32)
            n162 = Select(t="FAIL", s=w388, f="PASS") -> (s? t:f=→"IL_State":string)
            n163 = property on="IL_State" class="Str"("Text.TextColor"=w386) -> ()  [unwired: 2 in, 2 out]
          }
          frame "隔离" {
            n164 = Unbundle By Name(w403) -> ("ISL_State"=w407:bool)
            n165 = Or(x=w407, y=w406) -> (x .or. y?=w401:bool)
            n166 = Bundle By Name(cluster=w403, "ISL_State"=w401) -> (w402:T7)
            n167 = Select(t=u32 16711680 ("Text.Text Colors:Text Color"), s=w401, f=u32 6618880 ("Text.Text Colors:Text Color")) -> (s? t:f=w397:u32)
            n168 = Select(t="FAIL", s=w401, f="PASS") -> (s? t:f=→"ISL_State":string)
            n169 = property on="ISL_State" class="Str"("Text.TextColor"=w397) -> ()  [unwired: 2 in, 2 out]
          }
        }
      }
      frame "End_Test" {
        w409 = FALSE
        n170 = One Button Dialog(message="测试完成。") -> ()  [unwired: 1 in, 1 out]
        n171 = disable-structure shown="Disabled" {
          frame Disabled {
            w415 = ""
            n172 = local write "IL_State"(w415) -> ()
            n173 = local write "VSWR_State"(w415) -> ()
            n174 = local write "ISL_State"(w415) -> ()
          }
          frame Enabled {
          }
        }
        n175 = Bundle By Name(cluster=w412, "Index"=0, "VSWR_State"=w409, "IL_State"=w409, "ISL_State"=w409) -> (w410:T7)
      }
      frame "----------------------------" {
      }
      frame "Save" {
        n176 = call <vilib>:"Application Directory.vi"() -> ("Application Directory"=w422:path)
        n177 = Build Path(base path=w422, name or relative path=path "Config/Plot_Data") -> (appended path=w420:path)
        n178 = call "文件对话框"("start path"=w420, "prompt"="Plot_Data" ("default name"), "default name"="DUT ID:", "pattern (all files)"="*.xlsx;*.xls") -> ("selected path"=w424:path, "error out"=w423:errorcluster)  [unwired: 8 in, 2 out]
        n179 = case shown="No Error" w423 {
          tunnel: w424 -> [w432 _]
          frame No Error {
            w431 = TRUE ("close report? (T)")
            n180 = call <vilib>:"Application Directory.vi"() -> ("Application Directory"=w440:path)
            n181 = control-ref of="VSWR Graph"() -> (w447:refnum<vi>)
            n182 = control-ref of="IL Graph"() -> (w446:refnum<vi>)
            n183 = control-ref of="ISL Graph"() -> (w445:refnum<vi>)
            n184 = Build Path(base path=w440, name or relative path=path "Config/Plot_Template.xlsx") -> (appended path=w443:path)
            n185 = call <vilib>:"Create Report.vi"("window state (normal)"=T6."no change", "report type"=Report_Type."Excel", "template (empty)"=w443) -> ("report out"=w438:refnum<class "NI_report.lvclass">, "error out"=w435:errorcluster)  [unwired: 11 in]
            n186 = Build Array(w447, w446, w445) -> (w444:refnum<vi>[])
            n187 = for {
              tunnel: w444 -> [w456] mode=indexing
              shift-right: [w450] -> w437
              shift-left: w438 -> [w455]
              shift-right: [w449] -> w436
              shift-left: w435 -> [w448]
              i -> [w454]
              n188 = call "Write Graph to excel.vi"("Graph"=w456) -> ("excel data"=w451:string[][])  [unwired: 9 in, 1 out]
              n189 = call <vilib>:"Excel Get Worksheet.vi"("report in"=w455, "worksheet index (0)"=w454, "error in (no error)"=w448) -> ("report out"=w453:refnum<class "NI_report.lvclass">, "error out"=w452:errorcluster)  [unwired: 11 in]
              n190 = call-poly <vilib>:"Excel Easy Table.vi"("report in"=w453, "text data"=w451, "error in (no error)"=w452) -> ("report out"=w450:refnum<class "NI_report.lvclass">, "error out"=w449:errorcluster)  [unwired: 8 in, 3 out]
            }
            n191 = call-dynamic "Save Report to File.vi"("report in"=w437, "report file path"=w432, "error in (no error)"=w436) -> ("report out"=w433:refnum<class "NI_report.lvclass">, "error out"=w434:errorcluster)  [unwired: 11 in]
            n192 = call-dynamic "Dispose Report.vi"("report in"=w433, "wait until printing completed? (T)"=FALSE, "save changes? (F)"=w431, "error in (no error)"=w434, "close report? (T)"=w431) -> ()  [unwired: 10 in, 1 out]
          }
          frame Error {
          }
        }
      }
      frame "Load" {
        n193 = control-ref of="ISL Graph"() -> (w458:refnum<vi>)
        n194 = control-ref of="VSWR Graph"() -> (w460:refnum<vi>)
        n195 = control-ref of="IL Graph"() -> (w459:refnum<vi>)
        n196 = Build Array(w460, w459, w458) -> (w457:refnum<vi>[])
        n197 = call "Load Plot Data.vi"("Graph"=w457) -> ()  [unwired: 11 in]
      }
    }
    n198 = case shown="\"eee\", Default" w29 {
      selector: w29 -> [w35 _]
      tunnel: w32 -> [w39 w41]
      tunnel: w31 -> [w38 w40]
      tunnel: [w37 w40] -> w24
      tunnel: [w36 w41] -> _
      frame "eee", Default {
        n199 = Enqueue Element(queue=w39, element=w35, error in (no error)=w38) -> (queue out=w36:refnum<queue>, error out=w37:errorcluster)  [unwired: 1 in, 1 out]
      }
      frame "" {
      }
    }
  }
  n200 = while {
    tunnel: w8 -> [w466]
    tunnel: [w465] -> w10
    tunnel: w16 -> [w464]
    stop <- w467 stop-if-true
    n201 = event shown="[5] \"Save\": Value Change" {
      selector: w466 -> [_ _ _ _ _ _ _ _ _]
      dyn-events: [_ _ _ _ _ _ _ _ _] -> w465
      timeout: _ -> [_ _ _ _ _ _ _ _ _]
      tunnel: [_ _ _ _ _ _ _ w492 _] -> w467
      tunnel: w464 -> [_ _ w474 w477 w484 w487 w490 _ w496]
      event Timeout {
        n202 = event-data() -> ()  [unwired: 1 in, 1 out]
      }
      event Key Down {
        n203 = event-data() -> ("Char"=w469:i16, "PlatMods.Ctrl"=w468:bool)  [unwired: 1 in]
        n204 = case shown="True" w468 {
          tunnel: w469 -> [_ w470]
          frame False {
          }
          frame True {
            n205 = case shown="101" w470 {
              frame 0, Default {
              }
              frame 101 {
                n206 = property class="VI"("BDWin.Open"=TRUE ("程序框图窗口:打开")) -> ()  [unwired: 2 in, 2 out]
              }
            }
          }
        }
      }
      event Value Change {
        n207 = event-data() -> ()  [unwired: 1 in, 1 out]
        n208 = Unbundle By Name(w474) -> ("UI"=w473:refnum<queue>)
        n209 = Enqueue Element(queue=w473, element="Limit Line" ("元素")) -> ()  [unwired: 2 in, 3 out]
      }
      event "Panel Show": Value Change {
        n210 = event-data() -> ()  [unwired: 1 in, 1 out]
        n211 = Unbundle By Name(w477) -> ("UI"=w476:refnum<queue>)
        n212 = Enqueue Element(queue=w476, element="Panel Show" ("元素")) -> ()  [unwired: 2 in, 3 out]
      }
      event "Test": Value Change {
        n213 = event-data() -> ()  [unwired: 1 in, 1 out]
        n214 = Unbundle By Name(w484) -> ("UI"=w482:refnum<queue>)
        n215 = Enqueue Element(queue=w482, element="Clear Graph") -> (queue out=w480:refnum<queue>)  [unwired: 2 in, 2 out]
        n216 = Enqueue Element(queue=w480, element="Refresh Limit Line" ("元素")) -> (queue out=w478:refnum<queue>)  [unwired: 2 in, 2 out]
        n217 = Enqueue Element(queue=w478, element="Read_Switch_excel" ("元素")) -> ()  [unwired: 2 in, 3 out]
      }
      event "Save": Value Change {
        n218 = event-data() -> ()  [unwired: 1 in, 1 out]
        n219 = Unbundle By Name(w487) -> ("UI"=w486:refnum<queue>)
        n220 = Enqueue Element(queue=w486, element="Save" ("元素")) -> ()  [unwired: 2 in, 3 out]
      }
      event "Load": Value Change {
        n221 = event-data() -> ()  [unwired: 1 in, 1 out]
        n222 = Unbundle By Name(w490) -> ("UI"=w489:refnum<queue>)
        n223 = Enqueue Element(queue=w489, element="Load" ("元素")) -> ()  [unwired: 2 in, 3 out]
      }
      event User Event {
        n224 = event-data() -> ("Exit"=w493:string)  [unwired: 1 in]
        n225 = Equal?(x=w493, y="Exit") -> (x = y?=w492:bool)
      }
      event Panel Close? {
        n226 = event-data() -> ()  [unwired: 1 in, 1 out]
        n227 = Cluster To Array(cluster=w496) -> (array=w495:refnum<queue>[])
        n228 = for {
          tunnel: w495 -> [w499] mode=indexing
          tunnel: "Hide" ("元素") -> [w498]
          n229 = Enqueue Element(queue=w499, element=w498) -> ()  [unwired: 2 in, 3 out]
        }
        n230 = event-data("Discard?"=TRUE ("放弃？")) -> ()  [unwired: 1 in, 1 out]
      }
    }
  }
  n231 = Unregister For Events(event registration refnum=w10) -> (error out=w9:errorcluster)  [unwired: 1 in]
  n232 = Destroy User Event(user event=w11, error in=w9) -> (error out=w2:errorcluster)
  n233 = Merge Errors(w2, w1) -> (w6:errorcluster)
  n234 = Call Chain() -> (call chain=w4:string[])
  n235 = call <vilib>:"Clear Errors.vi"("error in (no error)"=w6) -> ("error out"=w5:errorcluster)  [unwired: 5 in, 1 out]
  n236 = Array Size(array=w4) -> (size(s)=w3:i32)
  n237 = case shown="2.." w3 {
    tunnel: w5 -> [_ w500]
    frame 0, Default {
    }
    frame 2.. {
      n238 = invoke class="VI" method="FP.Close"(error in=w500) -> ()  [unwired: 2 in, 3 out]
    }
  }
